vi "auto statelogger.vi"(8 "Rule name":string, 9 "Time":dbl format="%.2f", 10 "Plant State":T1=1 items=["OFF"], 11 "Datalog directory path":path) -> (0 "File Failure":bool)   [LabVIEW 2012]
uses:
  Plant state.ctl
  logic buffer cmd.ctl
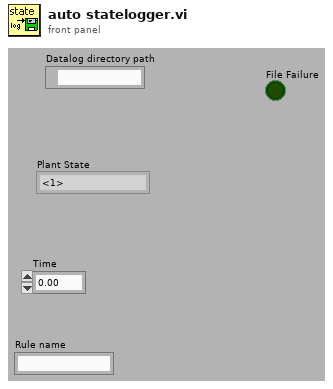
[diagram p1: front panel]
types:
  T1 = typedef "Plant state.ctl" = u16
  T2 = enum16{"open", "open or create", "create or replace", "create", "open (read only)"}
  T3 = typedef "logic buffer cmd.ctl" = enum16{"read", "write ouput settings", "write rules", "write setpoints", "write output descriptions", "write all", "calculate setpoints", "save", "open", "Load all setpoint code", "Load one setpoint code", "Configure one setpoint code"}
  T4 = typedef "rules.ctl" = T5[]
  T5 = typedef "State rules.ctl" = cluster{"state rules":T6[], "State name":string}
  T6 = typedef "rule.ctl" = cluster{"next state":u16, "conditions":T7[], "number of conditions":u8, "Rule name":string}
  T7 = typedef "condition.ctl" = cluster{"> or <":T8, "set point":i32, "sensors and variables":i32, "Data average interval":dbl}
  T8 = typedef "greater or less.ctl" = bool
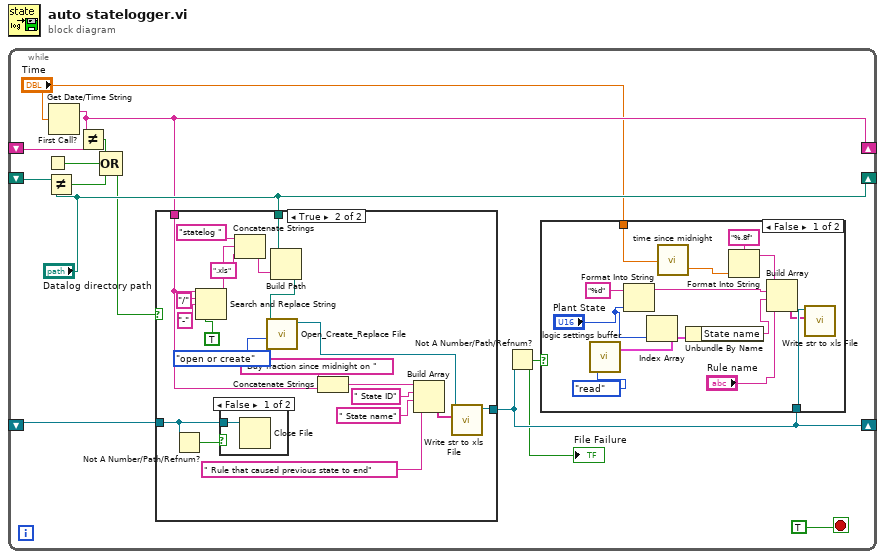
[diagram p0: block diagram]
diagram:
  n1 = while {
    shift-left: _ -> [w13]
    shift-right: ["Datalog directory path"] -> _
    shift-right: [w3] -> _
    shift-left: _ -> [w11]
    shift-right: [w6] -> _
    shift-left: _ -> [w5]
    stop <- TRUE stop-if-true
    n2 = First Call?() -> (First Call?: T/F=w9:bool)
    n3 = Not Equal?(x=w13, y="Datalog directory path") -> (x != y?=w8:bool)
    n4 = Get Date/Time String(seconds (now)="Time") -> (date string=w3:string)  [unwired: 2 in, 1 out]
    n5 = Not Equal?(x=w3, y=w11) -> (x != y?=w10:bool)
    n6 = Compound Arithmetic op=OR(w10, w9, w8) -> (w4:bool)
    n7 = case shown="True" w4 {
      tunnel: w5 -> [w14 w20]
      tunnel: [w14 w35] -> w6
      tunnel: "Datalog directory path" -> [_ w31]
      tunnel: w3 -> [_ w21]
      frame False {
      }
      frame True {
        n8 = Not A Number/Path/Refnum?(number/path/refnum=w20) -> (NaN/Path/Refnum?=w19:bool)
        n9 = Search and Replace String(replace all?=TRUE ("replace all? (F)"), input string=w21, search string="/", replace string="-" ("replace string (\"\")")) -> (result string=w28:string)  [unwired: 4 in, 3 out]
        n10 = case shown="False" w19 {
          tunnel: w20 -> [w36 _]
          frame False {
            n11 = Close File(refnum=w36) -> ()  [unwired: 1 in, 2 out]
          }
          frame True {
          }
        }
        n12 = Concatenate Strings("statelog " ("string"), w28, ".xls" ("string")) -> (w27:string)
        n13 = Build Path(base path=w31, name or relative path=w27) -> (appended path=w26:path)
        n14 = call <vilib>:"Open_Create_Replace File.vi"("function (open:0)"=T2."open or create", "file path"=w26) -> ("refnum"=w24:refnum<file>)  [unwired: 6 in, 3 out]
        n15 = Concatenate Strings("Day fraction since midnight on " ("Substring"), w21) -> (w23:string)
        n16 = Build Array(w23, " State ID" ("Substring"), " State name" ("Substring"), " Rule that caused previous state to end" ("Substring")) -> (w17:string[])
        n17 = call "Write str to xls File.vi"("1D data"=w17, "refnum"=w24) -> ("dup refnum"=w35:refnum<file>)  [unwired: 8 in, 1 out]
      }
    }
    n18 = Not A Number/Path/Refnum?(number/path/refnum=w6) -> (NaN/Path/Refnum?=w2:bool)
    "File Failure" <- w2
    n19 = case shown="False" w2 {
      tunnel: w6 -> [w50 _]
      tunnel: "Time" -> [w44 _]
      frame False {
        n20 = call "logic settings buffer.vi"("command"=logic_buffer_cmd."read") -> ("Rules out"=w41:T4)  [unwired: 11 in, 7 out]
        n21 = Format Into String(format string="%d", "Plant State") -> (resulting string=w46:string)  [unwired: 2 in, 1 out]
        n22 = Index Array(array=w41, index="Plant State") -> (element=w39:T5)
        n23 = call "time since midnight.vi"("seconds since 1Jan1904"=w44) -> ("Days"=w49:dbl)  [unwired: 1 out]
        n24 = Unbundle By Name(w39) -> ("State name"=w38:string)
        n25 = Format Into String(format string="%.8f" ("format (%.3f)"), w49) -> (resulting string=w45:string)  [unwired: 2 in, 1 out]
        n26 = Build Array(w45, w46, w38, "Rule name") -> (w43:string[])
        n27 = call "Write str to xls File.vi"("1D data"=w43, "refnum"=w50) -> ()  [unwired: 8 in, 2 out]
      }
      frame True {
      }
    }
  }
